vi "PM100D_FETCH.vi"(4 "error in":errorcluster, 7 "VISA in":refnum<visa-resource-name>="COM1") -> (0 "error out":errorcluster, 1 "Readout value":dbl format="%^#_9e", 2 "Readout string":string, 3 "VISA out":refnum<visa-resource-name>)   [LabVIEW 2014]
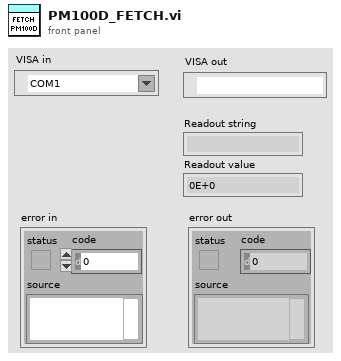
[diagram p1: front panel]
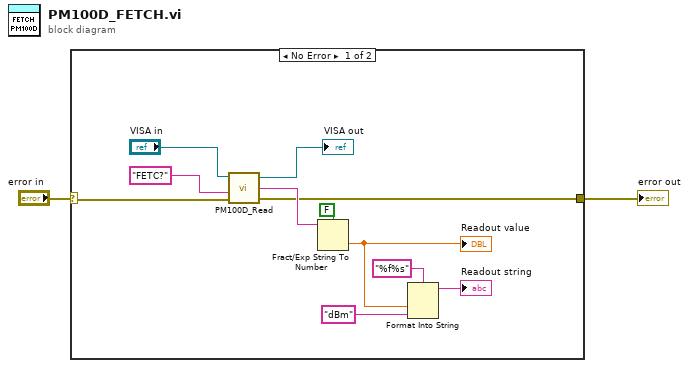
[diagram p0: block diagram]
diagram:
  n1 = case shown="No Error" "error in" {
    selector: "error in" -> [w6 w14]
    tunnel: [w5 w14] -> w1
    frame No Error {
      n2 = call "PM100D_Read.vi"("error in (no error)"=w6, "Command"="FETC?", "VISA in"="VISA in") -> ("error out"=w5:errorcluster, "ReadValue"=w12:string, "VISA out"=→"VISA out":refnum<visa-resource-name>)  [unwired: 1 in]
      n3 = Fract/Exp String To Number(use system decimal point (T)=FALSE, string=w12) -> (number=w9:dbl)  [unwired: 2 in, 1 out]
      "Readout value" <- w9
      n4 = Format Into String(format string="%f%s", w9, "dBm") -> (resulting string=→"Readout string":string)  [unwired: 2 in, 1 out]
    }
    frame Error {
    }
  }
  "error out" <- w1
